vi "Device Temperature.vi"(8 "error in (no error)":errorcluster, 10 "Device Temperature Arrays":T1) -> (0 "error out":errorcluster)   [LabVIEW 2015, in "Tool Module.lvlib"]
doc: "The arrays of device temperature sensors as well as the threshold values for controlling the cooling fan.\n_____\nCreated using Delacor QMH Event Scripter 3.1.0.29."
uses:
  Tool Module.lvlib
  Tool Typedefs/_Temperature All Arrays--typedef.ctl
  Device Temperature Argument--cluster.ctl
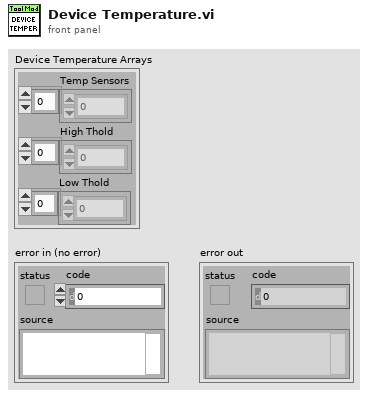
[diagram p1: front panel]
types:
  T1 = typedef "_Temperature All Arrays--typedef.ctl" = cluster{"Temp Sensors":dbl[], "High Thold ":dbl[], "Low Thold ":dbl[]}
  T2 = typedef "Tool Module.lvlib/Device Temperature Argument--cluster.ctl" = cluster{"Device Temperature Arrays":T1}
  T3 = typedef "Tool Module.lvlib/Broadcast Events--cluster.ctl" = cluster{"Module Did Init":refnum<user-event>, "Status Updated":refnum<user-event>, "Error Reported":refnum<user-event>, "Module Did Stop":refnum<user-event>, "Update Module Execution Status":refnum<user-event>, "Send Status":refnum<user-event>, "Trigger":refnum<user-event>, "Connected":refnum<user-event>, "Read from File Rtn":refnum<user-event>, "Device Temperature":refnum<user-event>}
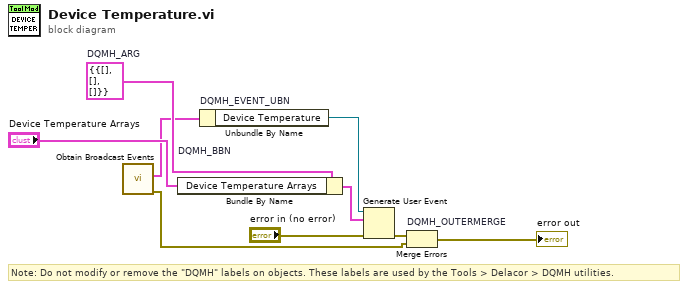
[diagram p0: block diagram]
diagram:
  w4 = T2 {"Device Temperature Arrays"={"Temp Sensors"=[], "High Thold "=[], "Low Thold "=[]}}  # DQMH_ARG
  # "Note: Do not modify or remove the \"DQMH\" labels on objects. These labels are used by the Tools > Delacor > DQMH utilities."
  n1 = call "Obtain Broadcast Events.vi"() -> ("error out"=w2:errorcluster, "Tool Module Broadcast Events"=w1:T3)  [unwired: 10 in]
  n2 = Bundle By Name "DQMH_BBN"(cluster=w4, "Device Temperature Arrays"="Device Temperature Arrays") -> (w7:T2)
  n3 = Unbundle By Name "DQMH_EVENT_UBN"(w1) -> ("Device Temperature"=w6:refnum<user-event>)
  n4 = Generate User Event(user event=w6, event data cluster=w7, error in="error in (no error)") -> (error out=w5:errorcluster)  [unwired: 1 in, 1 out]
  n5 = Merge Errors "DQMH_OUTERMERGE"(w5, w2) -> (→"error out":errorcluster)
